vi "Obtain Request Events.vi"(8 "error in":errorcluster, 10 "Create New? (F)":bool) -> (0 "error out":errorcluster, 2 "Sing Request Events":T1)   [LabVIEW 2024, in "Sing.lvlib"]
doc: "This VI Obtains/Creates the Requests events that will be used for other modules to communicate with the module that owns this VI. These Requests events will be accessed only via Public API methods for this module.\n\n<b>NOTE</b>: The contents of this VI are automatically generated and modified by the <b>Tools > DQMH Consortium > DQMH</b> utilities. Consider using those utilities instead of making your own modifications to this VI.\n_____\nBased on DQMH Dev Tools: Project Template 7.1.0.1503."
uses:
  Sing.lvlib
  Request Events--cluster.ctl
  Stop Argument--cluster.ctl
  Do Something Argument--cluster.ctl
  Do Something Else Argument--cluster.ctl
  Do Something Else and Wait for Reply Argument--cluster.ctl
  Do Something Else and Wait (Reply Payload)--cluster.ctl
  Show Panel Argument--cluster.ctl
  Hide Panel Argument--cluster.ctl
  Get Module Execution Status Argument--cluster.ctl
  Show Diagram Argument--cluster.ctl
  Change FP Color Argument--cluster.ctl
  Cambia de colores los paneles Argument--cluster.ctl
panel:
  # "NOTE: The contents of this VI are automatically generated and modified by the Tools > DQMH Consortium > DQMH utilities. Consider using those utilities instead of making your own modifications to this VI."
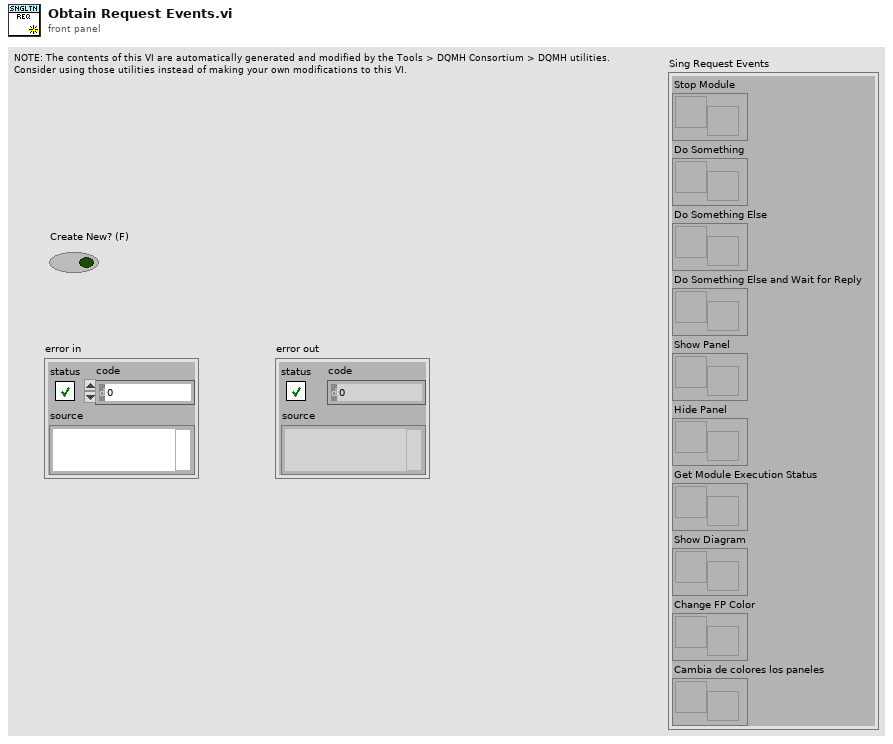
[diagram p1: front panel]
types:
  T1 = typedef "Sing.lvlib/Request Events--cluster.ctl" = cluster{"Stop Module":refnum<user-event>, "Do Something":refnum<user-event>, "Do Something Else":refnum<user-event>, "Do Something Else and Wait for Reply":refnum<user-event>, "Show Panel":refnum<user-event>, "Hide Panel":refnum<user-event>, "Get Module Execution Status":refnum<user-event>, "Show Diagram":refnum<user-event>, "Change FP Color":refnum<user-event>, "Cambia de colores los paneles":refnum<user-event>}
  T2 = typedef "Sing.lvlib/Cambia de colores los paneles Argument--cluster.ctl" = cluster{"Colores":u32[]}
  T3 = typedef "Sing.lvlib/Change FP Color Argument--cluster.ctl" = cluster{"FP Color":u32[]}
  T4 = typedef "Sing.lvlib/Hide Panel Argument--cluster.ctl" = cluster{"Hide Panel?":bool}
  T5 = typedef "Sing.lvlib/Show Panel Argument--cluster.ctl" = cluster{"Show Panel?":bool}
  T6 = typedef "Sing.lvlib/Show Diagram Argument--cluster.ctl" = cluster{"Debug?":bool}
  T7 = typedef "Sing.lvlib/Get Module Execution Status Argument--cluster.ctl" = cluster{"Running?":bool}
  T8 = typedef "Sing.lvlib/Do Something Else and Wait for Reply Argument--cluster.ctl" = cluster{"Do Something Else Msg":string, "X":dbl, "Wait Notifier":refnum<notifier>, "wait for reply":bool}
  T9 = typedef "Sing.lvlib/Do Something Else Argument--cluster.ctl" = cluster{"Do Something Else Msg":string, "X":dbl}
  T10 = typedef "Sing.lvlib/Do Something Argument--cluster.ctl" = cluster{"Do Something Msg":string}
  T11 = typedef "Sing.lvlib/Stop Argument--cluster.ctl" = cluster{"Origin":string, "Exit via Stop Module Req?":bool, "Wait for Module to stop?":bool}
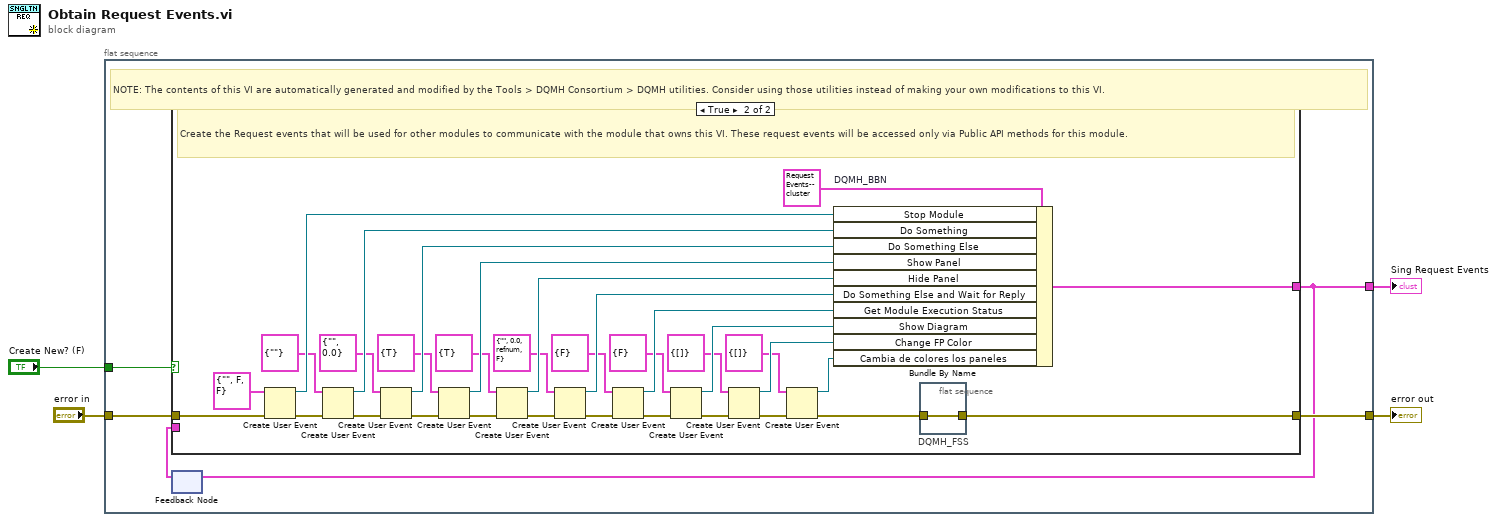
[diagram p0: block diagram]
diagram:
  n1 = flat-sequence {
    tunnel: [w9] -> w4
    tunnel: "error in" -> [w8]
    tunnel: [w6] -> w2
    tunnel: "Create New? (F)" -> [w5]
    frame #0 {
      # "NOTE: The contents of this VI are automatically generated and modified by the Tools > DQMH Consortium > DQMH utilities. Consider using those utilities instead of making your own modifications to this VI."
      n2 = feedback #1() -> (w7:T1)  [unwired: 1 in]
      n3 = case shown="True" w5 {
        tunnel: [w10 w26] -> w9
        tunnel: w8 -> [w10 w45]
        tunnel: [w11 w42] -> w6
        tunnel: w7 -> [w11 _]
        frame False {
          # "Obtain the Request events that were created in a previous call to this VI."
        }
        frame True {
          # "Create the Request events that will be used for other modules to communicate with the module that owns this VI. These request events will be accessed only via Public API methods for this module."
          n4 = Create User Event(user event datatype=T11 {"Origin"="", "Exit via Stop Module Req?"=FALSE, "Wait for Module to stop?"=FALSE} ("Stop Argument"), error in=w45) -> (user event=w43:refnum<user-event>, error out=w39:errorcluster)
          n5 = Create User Event(user event datatype=T10 {"Do Something Msg"=""} ("Do Something Argument"), error in=w39) -> (user event=w38:refnum<user-event>, error out=w37:errorcluster)
          n6 = Create User Event(user event datatype=T9 {"Do Something Else Msg"="", "X"=0.0} ("Do Something Else Argument"), error in=w37) -> (user event=w35:refnum<user-event>, error out=w34:errorcluster)
          n7 = Create User Event(user event datatype=T5 {"Show Panel?"=TRUE} ("Show Panel Argument"), error in=w34) -> (user event=w33:refnum<user-event>, error out=w32:errorcluster)
          n8 = Create User Event(user event datatype=T4 {"Hide Panel?"=TRUE} ("Hide Panel Argument"), error in=w32) -> (user event=w31:refnum<user-event>, error out=w30:errorcluster)
          n9 = Create User Event(user event datatype=T8 {"Do Something Else Msg"="", "X"=0.0, "Wait Notifier"=refnum, "wait for reply"=FALSE} ("Do Something Else and Wait for Reply Argument"), error in=w30) -> (user event=w29:refnum<user-event>, error out=w27:errorcluster)
          n10 = Create User Event(user event datatype=T7 {"Running?"=FALSE} ("Get Module Execution Status Argument"), error in=w27) -> (user event=w24:refnum<user-event>, error out=w25:errorcluster)
          n11 = Create User Event(user event datatype=T6 {"Debug?"=FALSE} ("Show Diagram Argument"), error in=w25) -> (user event=w21:refnum<user-event>, error out=w22:errorcluster)
          n12 = Create User Event(user event datatype=T3 {"FP Color"=[]} ("Change FP Color Argument"), error in=w22) -> (user event=w16:refnum<user-event>, error out=w17:errorcluster)
          n13 = Create User Event(user event datatype=T2 {"Colores"=[]} ("Cambia de colores los paneles Argument"), error in=w17) -> (user event=w13:refnum<user-event>, error out=w14:errorcluster)
          n14 = Bundle By Name "DQMH_BBN"(cluster=T1 {"Stop Module"=refnum, "Do Something"=refnum, "Do Something Else"=refnum, "Do Something Else and Wait for Reply"=refnum, "Show Panel"=refnum, "Hide Panel"=refnum, "Get Module Execution Status"=refnum, "Show Diagram"=refnum, "Change FP Color"=refnum, "Cambia de colores los paneles"=refnum} ("output cluster"), "Stop Module"=w43, "Do Something"=w38, "Do Something Else"=w35, "Show Panel"=w33, "Hide Panel"=w31, "Do Something Else and Wait for Reply"=w29, "Get Module Execution Status"=w24, "Show Diagram"=w21, "Change FP Color"=w16, "Cambia de colores los paneles"=w13) -> (w42:T1)
          n15 = flat-sequence "DQMH_FSS" {
            tunnel: w14 -> [w46]
            tunnel: [w46] -> w26
            frame #0 {
            }
          }
        }
      }
      n16 = feedback-in #1(w6) -> ()
    }
  }
  "Sing Request Events" <- w2
  "error out" <- w4
